vi "PH_Cont-601k_PSU.evt Call Set Configuration.vi"(0 "i ref in":refnum<vi>, 1 "Instance name":string="N/A", 4 "Configuration to set":T1 items=["Ch intl, Fl intl, QSw intl", "Ch intl, Fl intl, QSw ext", "Ch intl, Fl ext, QSw intl", "Ch intl, Fl ext, QSw ext", "Ch ext, Fl int, QSw int", "Ch ext, Fl int, QSw ext", "Ch ext, Fl ext, QSw int", "Ch ext, Fl ext, QSw ext"], 5 "error in":errorcluster) -> (14 "i ref out":refnum<vi>, 19 "error out":errorcluster)   [LabVIEW 2014, in "PH_Cont-601k_PSU.lvlib"]
doc: "This VI calls an event by a simple call."
uses:
  PH_Cont-601k_PSU.lvlib
  PH_Cont-601k_PSU.Configuration.ctl
  CSCore/CSSystem/CoreLib/CoreLib.short 2 byte array.vi
  CSCore/BaseProcess/BaseProcess.lvlib
  CSCore/CSSystem/CoreLib/CoreLib.lvlib
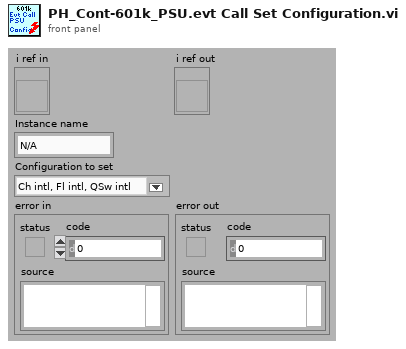
[diagram p1: front panel]
types:
  T1 = typedef "PH_Cont-601k_PSU.lvlib/PH_Cont-601k_PSU.Configuration.ctl" = u16
  T2 = typedef "CoreDefs.rawDataType.ctl" = i8[]
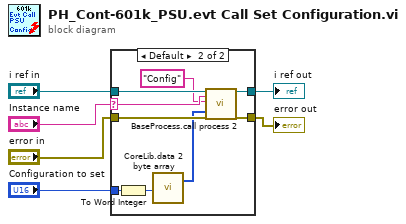
[diagram p0: block diagram]
diagram:
  n1 = case shown="Default" "Instance name" {
    selector: "Instance name" -> [_ w13]
    tunnel: [w7 w17] -> w6
    tunnel: "error in" -> [w7 w16]
    tunnel: [w8 w15] -> w3
    tunnel: "i ref in" -> [w8 w14]
    tunnel: "Configuration to set" -> [_ w10]
    frame "", "N/A" {
    }
    frame Default {
      n2 = To Word Integer(number=w10) -> (16bit integer=w9:i16)
      n3 = call-poly "CoreLib.data 2 byte array.vi"("i16"=w9) -> ("byteArray out"=w11:T2)  [unwired: 18 in]
      n4 = call "BaseProcess.call process 2.vi"("i ref in"=w14, "Object"=w13, "Selector"="Config", "Data"=w11, "error in (no error)"=w16) -> ("i ref out"=w15:refnum<vi>, "error out"=w17:errorcluster)  [unwired: 13 in]
    }
  }
  "error out" <- w6
  "i ref out" <- w3
